vi "Read configuration.vi"(8 "error in":errorcluster, 11 "SQLite editor node in":refnum<class "SQLite editor node.lvclass">) -> (0 "error out":errorcluster, 2 "configuration":refnum<class "NISE_CEF_serializable configuration.lvclass">, 3 "SQLite editor node out":refnum<class "SQLite editor node.lvclass">)   [LabVIEW 2014, in "SQLite editor node.lvclass"]
uses:
  SQLite editor node.lvclass
  <vilib>/NI/Configuration Framework/serializable configuration/NISE_CEF_serializable configuration.lvclass
  SQLite editor node.lvclass/SQLite editor node.ctl
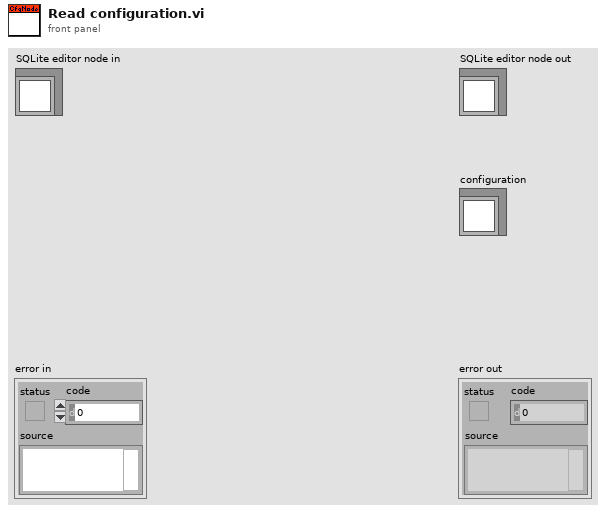
[diagram p1: front panel]
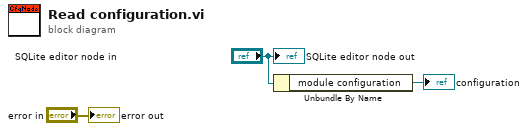
[diagram p0: block diagram]
diagram:
  n1 = Unbundle By Name("SQLite editor node in") -> ("module configuration"=→"configuration":refnum<class "SQLite configuration.lvclass">)
  "error out" <- "error in"
  "SQLite editor node out" <- "SQLite editor node in"
